vi "LAOnError.vi"(8 "Error In":errorcluster, 11 "LiteAgent In":T1) -> (0 "Error Out":errorcluster, 2 "ErrorMessage":string, 3 "LiteAgent Out":T1)   [LabVIEW 2017, in "LiteAgentSDK.lvlib"]
uses:
  LiteAgentSDK.lvlib
  C:/Users/Jan/Projects/LiteAgentSDK-LabVIEW/Source/Bin/LiteAgentSDK.LabVIEW.dll
  Bin/LiteAgentSDK.LabVIEW.dll
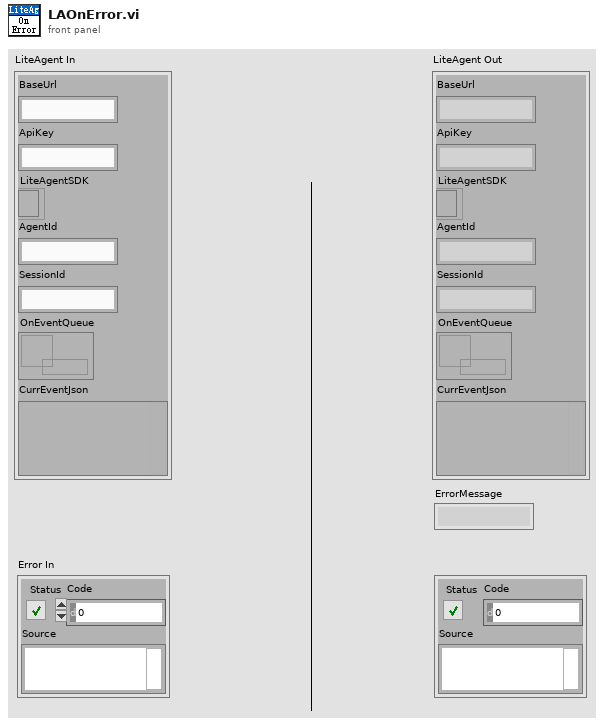
[diagram p1: front panel]
types:
  T1 = cluster{"BaseUrl":string, "ApiKey":string, "LiteAgentSDK":refnum<k24>, "AgentId":string, "SessionId":string, "OnEventQueue":refnum<queue>, "CurrEventJson":variant}
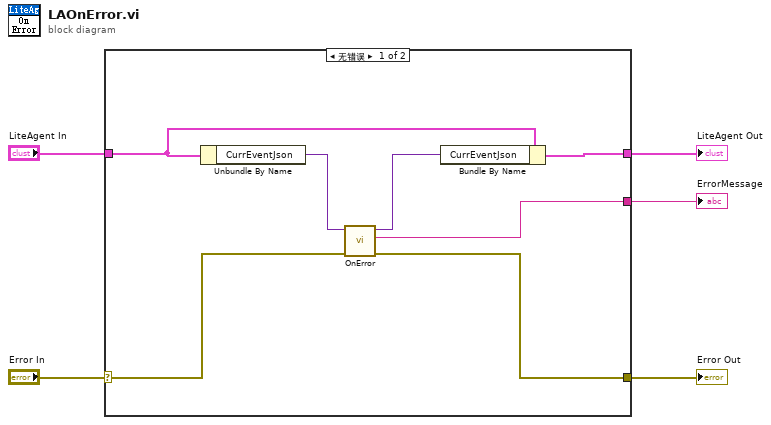
[diagram p0: block diagram]
diagram:
  n1 = case shown="无错误" "Error In" {
    selector: "Error In" -> [w9 w14]
    tunnel: [w8 w14] -> w4
    tunnel: "LiteAgent In" -> [w12 w13]
    tunnel: [w11 w13] -> w2
    tunnel: [w6 _] -> w1
    frame No Error {
      n2 = Unbundle By Name(w12) -> ("CurrEventJson"=w10:variant)
      n3 = call "OnError.vi"("Error In"=w9, "JSON Tree In"=w10) -> ("Error Out"=w8:errorcluster, "Message"=w6:string, "JSON Tree Out"=w7:variant)  [unwired: 7 in]
      n4 = Bundle By Name(cluster=w12, "CurrEventJson"=w7) -> (w11:T1)
    }
    frame Error {
    }
  }
  "Error Out" <- w4
  "LiteAgent Out" <- w2
  "ErrorMessage" <- w1
